vi "QAM Components.vi"(0 "FFT Downsampled":cdb[](array[numeric])) -> (1 "FFT , Data":cdb[](array[numeric]), 2 "FFT , Pilot":cdb[](array[numeric]))   [LabVIEW 2018]
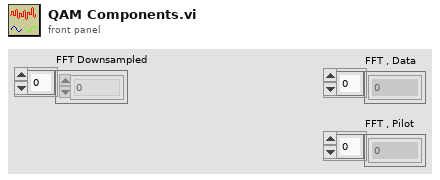
[diagram p1: front panel]
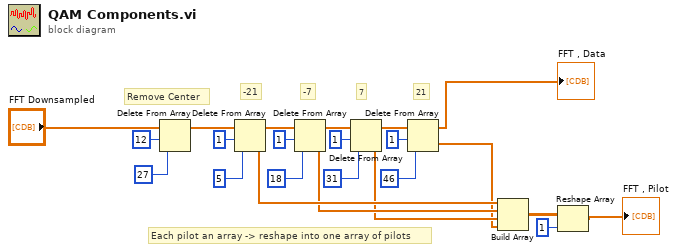
[diagram p0: block diagram]
diagram:
  # "Each pilot an array -> reshape into one array of pilots"
  # "21"
  # "7"
  # "-7"
  # "-21"
  # "Remove Center"
  n1 = Delete From Array(array="FFT Downsampled", length=12, index=27) -> (array with subset deleted=w20:cdb[])  [unwired: 1 out]
  n2 = Delete From Array(array=w20, length=1, index=5) -> (deleted portion=w7:cdb[], array with subset deleted=w15:cdb[])
  n3 = Delete From Array(array=w15, length=1, index=18) -> (deleted portion=w6:cdb[], array with subset deleted=w12:cdb[])
  n4 = Delete From Array(array=w12, length=1, index=31) -> (deleted portion=w5:cdb[], array with subset deleted=w9:cdb[])
  n5 = Delete From Array(array=w9, length=1, index=46) -> (deleted portion=w4:cdb[], array with subset deleted=→"FFT , Data":cdb[])
  n6 = Build Array(w7, w6, w5, w4) -> (w3:cdb[][])
  n7 = Reshape Array(w3, 1 ("dimension size")) -> (→"FFT , Pilot":cdb[])
